vi "Globale Variablen.vi"() -> ()   [LabVIEW 2024]
panel:
  in  "Kamera Unten n.i.O.":bool
  in  "ACK SPS":bool
  in  "Kontakt zu groß":bool
  in  "Referenzen nicht gefunden":bool
  in  "Kontakt zu klein":bool
  in  "Referenzen nicht in Lichtgitter":bool
  in  "Kontaktposition nicht gefunden":bool
  in  "Kontaktnummer in":i16
  in  "Position in y":sgl
  in  "Position in x":sgl
  in  "Vermessung Lichtgitter fertig":bool
  in  "Nachkontrolle Kamera Unten fertig":bool
  in  "Koordinaten ermittelt":bool
  in  "Fehler SPS":bool
  in  "Fehler Lichtgitter":bool
  in  "Fehler Flüssiglinse":bool
  in  "Fehler Kamera Unten":bool
  in  "Fehler Kamera Oben":bool
  in  "Betriebsart SPS":T1(ring)
  in  "Pneumatik OK":bool
  in  "Türen OK":bool
  in  "NOT-HALT":bool
  in  "Lebensbit SPS":bool
  in  "Automatik läuft":bool
  in  "Störung SPS":bool
  in  "Richten LabVIEW":bool
  in  "LabVIEW Bereit":bool
  in  "Störung LabVIEW":bool
  in  "Lebensbit LabVIEW":bool
  out "Winkle Kontakt":dbl
  in  "Fertigungsauftrag":string
  out "Position y":dbl
  out "Position x":dbl
  out "Offset y":dbl
  out "Offset x":dbl
  in  "Artikeldaten von SPS laden":bool
  in  "Belichtungszeiten & Fokus":dbl[](array[numeric])
  in  "Start Vermessung Lichtgitter":bool
  in  "Kontaktanzahl":u32
  in  "Kontaktpositionen":cluster{"Abstand":dbl, "Winkel":dbl}[](array[cluster])
  in  "Artikelnummer":string
  in  "Start Nachkontrolle Kamera Unten":bool
  in  "Start Koordinaten ermitteln":bool
  out "Fehlermeldung SPS":errorcluster
  in  "SPS neu verbinden":bool
  in  "Programm beenden":bool
  # "SPS"
  # "LabVIEW"
  # "IN"
  # "OUT"
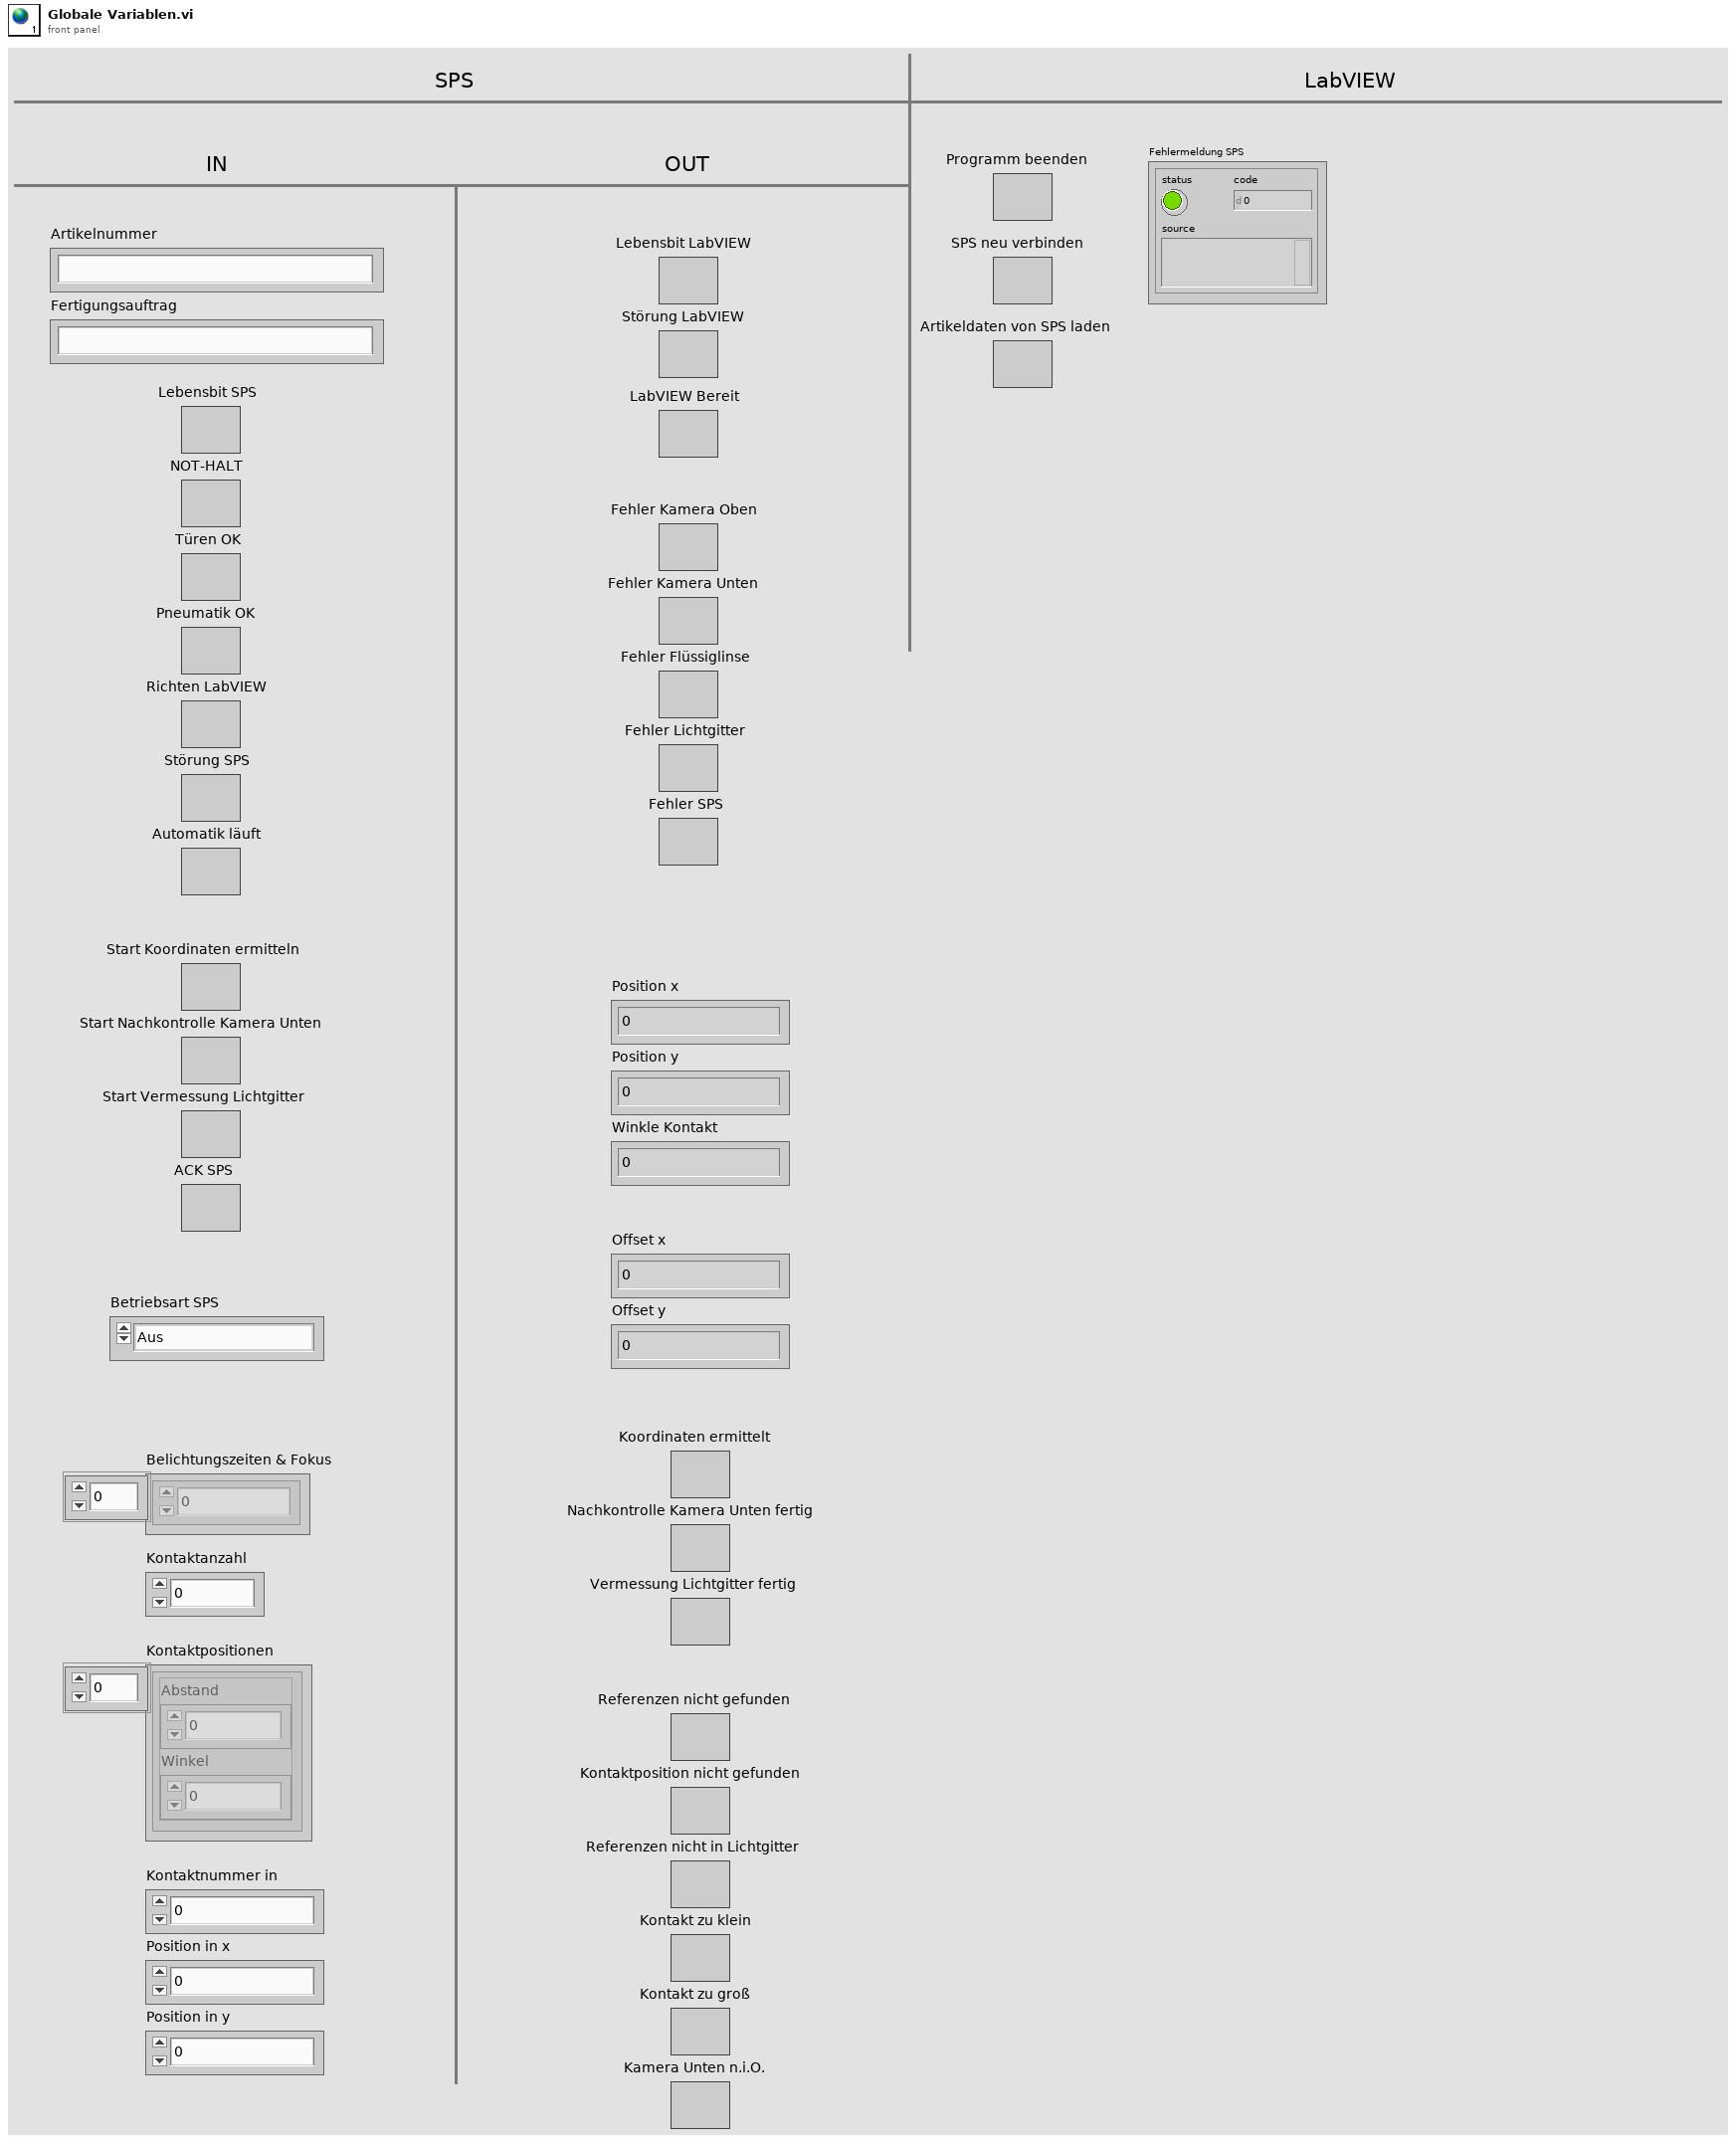
[diagram p1: front panel]
types:
  T1 = enum16{"Aus", "Manuell", "Automatik", "Verwaltung", "Richten"}
diagram:
